vi "PGselect.vi"(8 "error in":errorcluster, 11 "conn":u32) -> (0 "error out":errorcluster, 2 "Data":string[](array[string]), 3 "conn_out":u32)   [LabVIEW 2019]
uses:
  libpqlv/libpqlv.lvlib
  libpqutility.lvlib
panel:
  out "PQsendQuery":i32
  out "PQresultStatus":T1(ring)
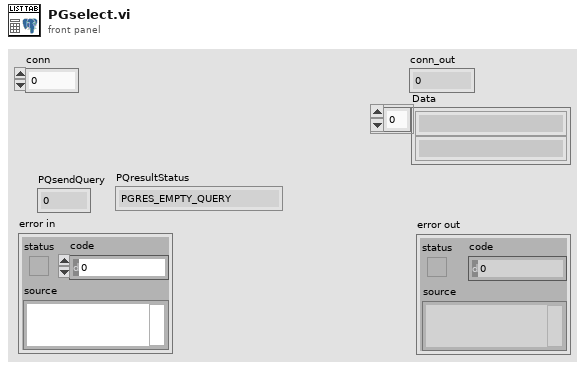
[diagram p1: front panel]
types:
  T1 = enum16{"PGRES_EMPTY_QUERY", "PGRES_COMMAND_OK", "PGRES_TUPLES_OK", "PGRES_COPY_OUT", "PGRES_COPY_IN", "PGRES_BAD_RESPONSE", "PGRES_NONFATAL_ERROR", "PGRES_FATAL_ERROR"}
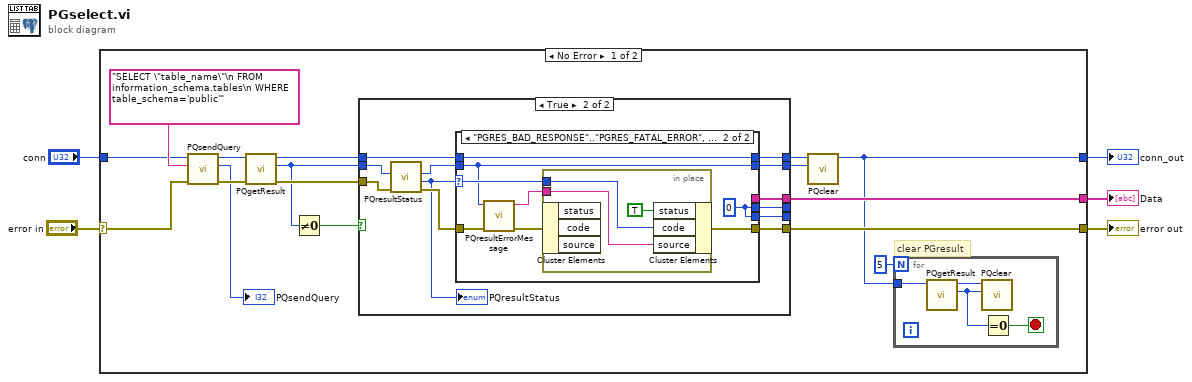
[diagram p0: block diagram]
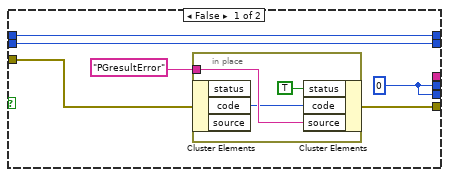
[diagram p2: hidden frame]
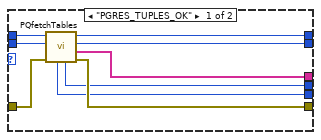
[diagram p3: hidden frame]
diagram:
  n1 = case shown="No Error" "error in" {
    selector: "error in" -> [w11 w68]
    tunnel: "conn" -> [w12 w67]
    tunnel: [w13 w68] -> w4
    tunnel: [w6 w67] -> w2
    tunnel: [w10 _] -> w1
    frame No Error {
      # "clear PGresult"
      n2 = call "PQsendQuery.vi"("error in (no error)"=w11, "query"="SELECT \"table_name\"\n FROM information_schema.tables\n WHERE table_schema='public'", "conn"=w12) -> ("error out"=w21:errorcluster, "PQsendQuery"=→"PQsendQuery":i32, "conn_out"=w9:u32)  [unwired: 6 in]
      n3 = call "PQgetResult.vi"("error in (no error)"=w21, "conn"=w9) -> ("error out"=w20:errorcluster, "PGresult"=w19:u32, "conn_out"=w8:u32)  [unwired: 7 in]
      n4 = Not Equal To 0?(x=w19) -> (x != 0?=w18:bool)
      n5 = case shown="True" w18 {
        tunnel: w20 -> [w25 w42]
        tunnel: w8 -> [w22 w41]
        tunnel: [_ w39] -> w10
        tunnel: [w27 w38] -> _
        tunnel: [w24 w37] -> w13
        tunnel: w19 -> [w26 w35]
        tunnel: [w27 w36] -> _
        tunnel: [w26 w33] -> w14
        tunnel: [w22 w31] -> w7
        frame False {
          w27 = u32 0 ("PQnTuples")
          n6 = in-place {
            in-place-border: "PGresultError" ("source") -> [w30]
            n7 = in-place-cluster #1(w25) -> ("code"=w28:i32)  [unwired: 2 out]
            n8 = in-place-cluster #1("status"=TRUE, "code"=w28, "source"=w30) -> (w24:errorcluster)
          }
        }
        frame True {
          n9 = call "PQresultStatus.vi"("error in (no error)"=w42, "res"=w35) -> ("error out"=w40:errorcluster, "PQresultStatus"=w34:T1, "res out"=w32:u32)  [unwired: 7 in]
          "PQresultStatus" <- w34
          n10 = case shown="\"PGRES_BAD_RESPONSE\"..\"PGRES_FATAL_ERROR\", Default" w34 {
            selector: w34 -> [_ w55]
            tunnel: w32 -> [w50 w53]
            tunnel: [w44 w58] -> w38
            tunnel: w40 -> [w51 w59]
            tunnel: w41 -> [w49 w52]
            tunnel: [w48 _] -> w39
            tunnel: [w45 w54] -> w37
            tunnel: [w43 w58] -> w36
            tunnel: [w47 w53] -> w33
            tunnel: [w46 w52] -> w31
            frame "PGRES_TUPLES_OK" {
              n11 = call "PQfetchTables.vi"("error in"=w51, "res"=w50, "conn"=w49) -> ("error out"=w45:errorcluster, "Data"=w48:string[], "res_out"=w47:u32, "conn_out"=w46:u32, "PQnTuples"=w44:i32, "PQnFields"=w43:i32)  [unwired: 3 in]
            }
            frame "PGRES_BAD_RESPONSE".."PGRES_FATAL_ERROR", Default {
              w58 = u32 0 ("PQnTuples")
              n12 = call "PQresultErrorMessage.vi"("error in (no error)"=w59, "res"=w53) -> ("error out"=w56:errorcluster, "PQresultErrorMessage"=w57:string)  [unwired: 8 in]
              n13 = in-place {
                in-place-border: w57 -> [w62]
                in-place-border: w55 -> [w60]
                n14 = in-place-cluster #2(w56) -> ()  [unwired: 3 out]
                n15 = in-place-cluster #2("status"=TRUE, "code"=w60, "source"=w62) -> (w54:errorcluster)
              }
            }
          }
        }
      }
      n16 = call "PQclear.vi"("res"=w14, "conn"=w7) -> ("conn_out"=w6:u32)  [unwired: 8 in, 1 out]
      n17 = for {
        N: 5 -> [_]
        tunnel: w6 -> [w63]
        stop <- w65 stop-if-true
        n18 = call "PQgetResult.vi"("conn"=w63) -> ("PGresult"=w64:u32, "conn_out"=w66:u32)  [unwired: 8 in, 1 out]
        n19 = call "PQclear.vi"("res"=w64, "conn"=w66) -> ()  [unwired: 8 in, 2 out]
        n20 = Equal To 0?(x=w64) -> (x = 0?=w65:bool)
      }
    }
    frame Error {
    }
  }
  "conn_out" <- w2
  "error out" <- w4
  "Data" <- w1
